vi "CIMAQ Overlay Points Big.vi"(0 "Image In":T1, 1 "Point":cluster{"X":i32, "Y":i32}, 2 "Overlay Thickness":i32(slide)=5 scale=0.0..20.0, 3 "error in (no error)":errorcluster, 4 "Color":u32(colorbox)=16711680) -> (7 "Image Out":T1, 10 "error out":errorcluster)   [LabVIEW 2014]
uses:
  <vilib>/vision/Image Controls.llb/IMAQ Image.ctl
panel:
  in  "OverlayName":string="test"
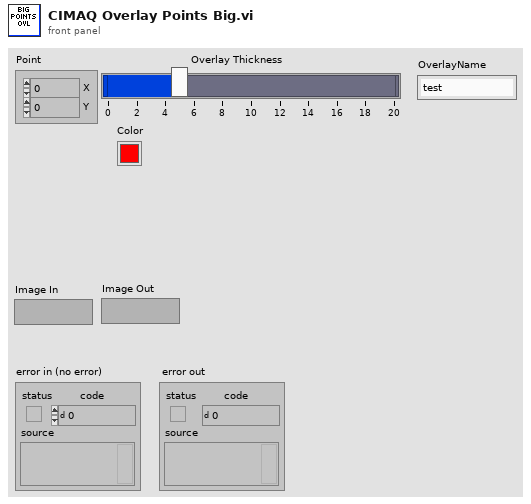
[diagram p1: front panel]
types:
  T1 = typedef "IMAQ Image.ctl" = refnum<image>
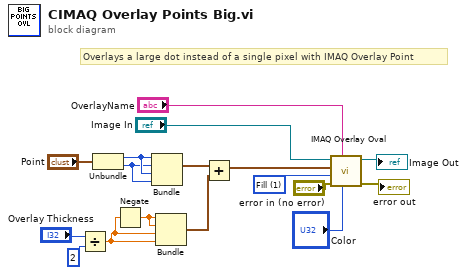
[diagram p0: block diagram]
diagram:
  w3 = u32 1 items=["Frame", "Fill"] ("Drawing Mode (Frame)")
  # "Overlays a large dot instead of a single pixel with IMAQ Overlay Point"
  n1 = Divide(x="Overlay Thickness", y=2) -> (x/y=w12:dbl)
  n2 = Unbundle("Point") -> ("X"=w9:i32, "Y"=w8:i32)
  n3 = Negate(x=w12) -> (-x=w11:dbl)
  n4 = Bundle("X"=w9, "Y"=w8, "X"=w9, "Y"=w8) -> (w7:cluster{"X":i32, "Y":i32, "X":i32, "Y":i32})  [unwired: 1 in]
  n5 = Bundle(w11, w11, w12, w12) -> (w6:cluster{dbl, dbl, dbl, dbl})  [unwired: 1 in]
  n6 = Add(x=w7, y=w6) -> (x+y=w5:cluster{dbl, dbl, dbl, dbl})
  n7 = call "IMAQ Overlay Oval"("Color"="Color", "Group"="OverlayName", "error in (no error)"="error in (no error)", "Drawing Mode (Frame)"=w3, "Bounding Rectangle"=w5, "Image"="Image In") -> ("error out"=→"error out":errorcluster, "Image Out"=→"Image Out":T1)  [unwired: 4 in]
